vi "Get VI Settings - Method Options - Options.vi"(8 "error in (no error)":errorcluster {"code" format="Error %.0f"}, 11 "VIDoc Printer In":refnum<class "VIDoc Printer.lvclass">) -> (0 "error out":errorcluster {"code" format="Error %.0f"}, 2 "Options":bool=TRUE, 3 "VIDoc Printer Out":refnum<class "VIDoc Printer.lvclass">)   [LabVIEW 2023, in "VIDoc Printer.lvlib" / "VIDoc Printer.lvclass"]
uses:
  VIDoc Printer.lvclass
  VIDoc Printer.lvclass/VIDoc Printer.ctl
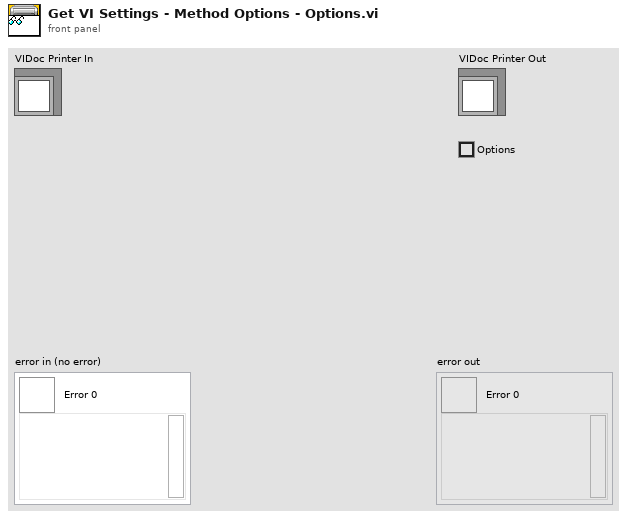
[diagram p1: front panel]
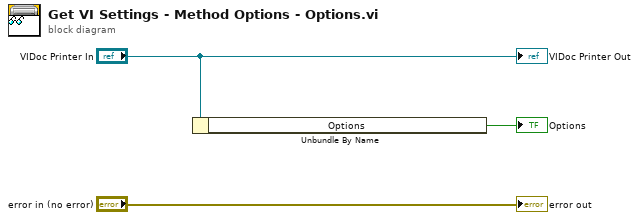
[diagram p0: block diagram]
diagram:
  n1 = Unbundle By Name("VIDoc Printer In") -> ("Options"=→"Options":bool)
  "error out" <- "error in (no error)"
  "VIDoc Printer Out" <- "VIDoc Printer In"
